vi "FRCts20_Backend_GenerateStats.vi"(8 "error in (no error)":errorcluster, 9 "Key":string, 11 "TeamData":T1) -> (0 "error out":errorcluster)   [LabVIEW 2014, in "FRCts20_Backend_Engine_Deprecated.lvlib"]
uses:
  FRCts20_Backend_Engine_Deprecated.lvlib
  FRCts20_Backend_NumTeams.ctl
  FRCts20_Backend_Controls.lvlib
  FRCts20_Backend_PercTeams.ctl
  FRCts20_Backend_SoftwareUsage.ctl
  FRCts20_Backend_ResPerDayPerQuad.ctl
  FRCts20_Backend_ResDayTotals.ctl
  FRCts20_Backend_ResQuadTotals.ctl
  FRCts20_Backend_Resolved.ctl
  FRCts20_Backend_OpenQuadTotals.ctl
  FRCts20_Backend_Open.ctl
  FRCts20_Backend_Issues.ctl
  FRCts20_Backend_Stats.ctl
  FRCts20_Backend_Engine.lvlib
  FRCts20_Backend_FGVOperation.ctl
  FRCts20_Backend_FGVDatesCommands.ctl
  FRCts20_Backend_IssueDfn.ctl
  FRCts20_Backend_TeamDfn.ctl
  FRCts20_Backend_TeamDataDfn.ctl
  FRCts20_Backend_Team_Info.ctl
  FRCts20_Backend_Note.ctl
  FRCts20_Backend_Note_list.ctl
  FRCts20_Backend_request_info.ctl
  FRCts20_Backend_IssueTeamList.ctl
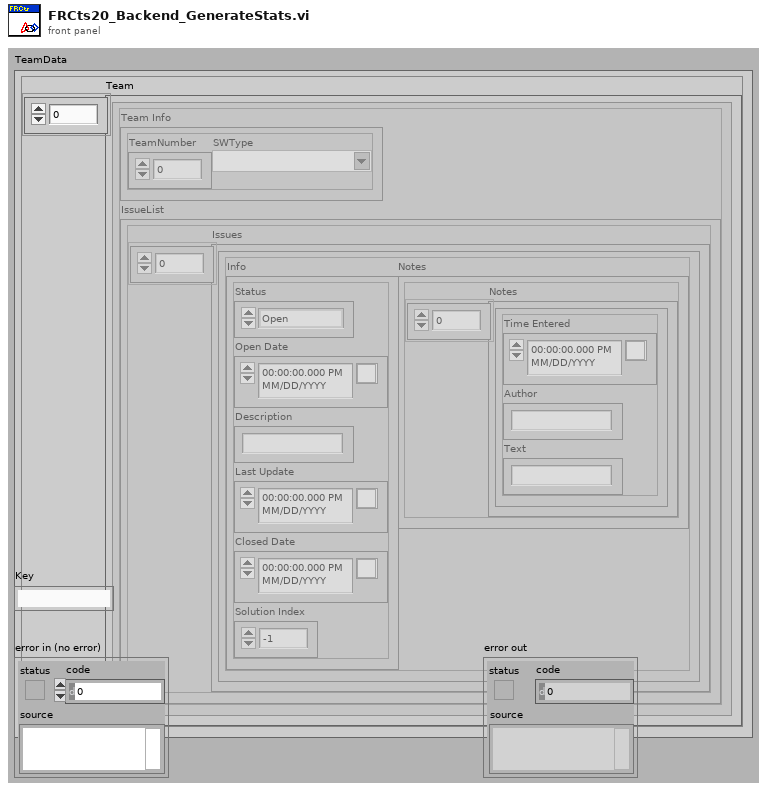
[diagram p1: front panel]
types:
  T1 = typedef "FRCts20_Backend_Controls.lvlib/FRCts20_Backend_TeamDataDfn.ctl" = cluster{"Team":T2[]}
  T2 = typedef "FRCts20_Backend_Controls.lvlib/FRCts20_Backend_TeamDfn.ctl" = cluster{"Team Info":T3, "IssueList":T4}
  T3 = typedef "FRCts20_Backend_Controls.lvlib/FRCts20_Backend_Team_Info.ctl" = cluster{"TeamNumber":u16, "SWType":string}
  T4 = typedef "FRCts20_Backend_Controls.lvlib/FRCts20_Backend_IssueTeamList.ctl" = cluster{"Issues":T5[]}
  T5 = typedef "FRCts20_Backend_Controls.lvlib/FRCts20_Backend_IssueDfn.ctl" = cluster{"Notes":T6, "Info":T8}
  T6 = typedef "FRCts20_Backend_Controls.lvlib/FRCts20_Backend_Note_list.ctl" = cluster{"Notes":T7[]}
  T7 = typedef "FRCts20_Backend_Controls.lvlib/FRCts20_Backend_Note.ctl" = cluster{"Time Entered":timestamp, "Author":string, "Text":string}
  T8 = typedef "FRCts20_Backend_Controls.lvlib/FRCts20_Backend_request_info.ctl" = cluster{"Status":enum16{"Open", "In Work", "Closed"}, "Open Date":timestamp, "Description":string, "Last Update":timestamp, "Closed Date":timestamp, "Solution Index":i32}
  T9 = typedef "FRCts20_Backend_Engine.lvlib/FRCts20_Backend_FGVOperation.ctl" = enum16{"Initialize", "EnqueueMessage", "EnqueueDataReturn", "FlushMessage", "FlushDataReturn"}
  T10 = typedef "FRCts20_Backend_Controls.lvlib/FRCts20_Backend_FGVDatesCommands.ctl" = enum16{"Set Dates", "Get Day", "Get First Day"}
  T11 = typedef "FRCts20_Backend_Controls.lvlib/FRCts20_Backend_Stats.ctl" = cluster{"SoftwareUsage":T12, "Issues":T15}
  T12 = typedef "FRCts20_Backend_Controls.lvlib/FRCts20_Backend_SoftwareUsage.ctl" = cluster{"NumTeams":T13, "PercTeams":T14}
  T13 = typedef "FRCts20_Backend_Controls.lvlib/FRCts20_Backend_NumTeams.ctl" = cluster{"LabVIEW_Num":u16, "C_Cpp_Num":u16, "Java_Num":u16, "Other_Num":u16}
  T14 = typedef "FRCts20_Backend_Controls.lvlib/FRCts20_Backend_PercTeams.ctl" = cluster{"LabVIEW_Perc":dbl, "C_Cpp_Perc":dbl, "Java_Perc":dbl, "Other_Perc":dbl}
  T15 = typedef "FRCts20_Backend_Controls.lvlib/FRCts20_Backend_Issues.ctl" = cluster{"Resolved":T16, "Open":T20}
  T16 = typedef "FRCts20_Backend_Controls.lvlib/FRCts20_Backend_Resolved.ctl" = cluster{"Total":u16, "AvgTimeRes":dbl, "PerDayPerQuad":T17, "DayTotals":T18, "QuadTotals":T19}
  T17 = typedef "FRCts20_Backend_Controls.lvlib/FRCts20_Backend_ResPerDayPerQuad.ctl" = cluster{"Day1Quad1":u16, "Day1Quad2":u16, "Day1Quad3":u16, "Day1Quad4":u16, "Day2Quad1":u16, "Day2Quad2":u16, "Day2Quad3":u16, "Day2Quad4":u16, "Day3Quad1":u16, "Day3Quad2":u16, "Day3Quad3":u16, "Day3Quad4":u16, "Day4Quad1":u16, "Day4Quad2":u16, "Day4Quad3":u16, "Day4Quad4":u16}
  T18 = typedef "FRCts20_Backend_Controls.lvlib/FRCts20_Backend_ResDayTotals.ctl" = cluster{"Day1":u16, "Day2":u16, "Day3":u16, "Day4":u16}
  T19 = typedef "FRCts20_Backend_Controls.lvlib/FRCts20_Backend_ResQuadTotals.ctl" = cluster{"Quad1":u16, "Quad2":u16, "Quad3":u16, "Quad4":u16}
  T20 = typedef "FRCts20_Backend_Controls.lvlib/FRCts20_Backend_Open.ctl" = cluster{"Total":u16, "QuadTotals":T21}
  T21 = typedef "FRCts20_Backend_Controls.lvlib/FRCts20_Backend_OpenQuadTotals.ctl" = cluster{"Quad1":u16, "Quad2":u16, "Quad3":u16, "Quad4":u16}
  T22 = cluster{"LabVIEW_Num":dbl, "C_Cpp_Num":dbl, "Java_Num":dbl, "Other_Num":dbl}
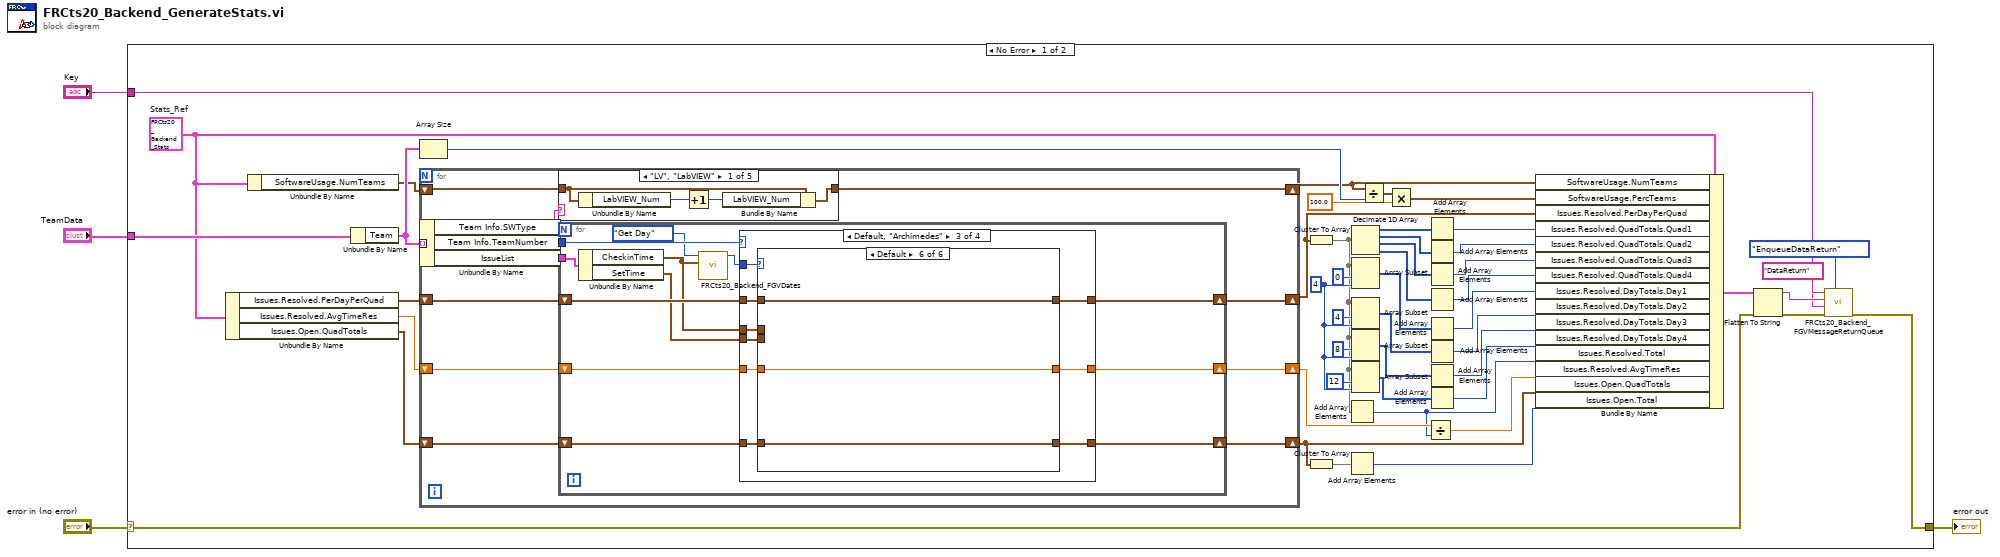
[diagram p0: block diagram]
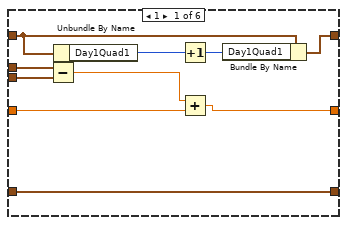
[diagram p3: hidden frame]
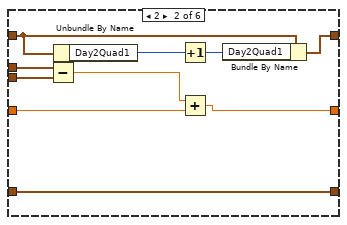
[diagram p4: hidden frame]
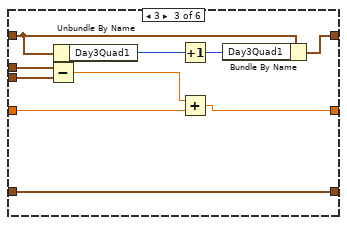
[diagram p5: hidden frame]
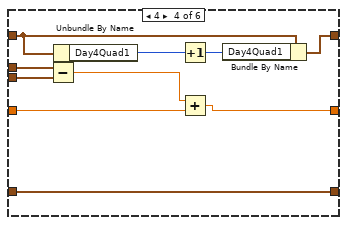
[diagram p6: hidden frame]
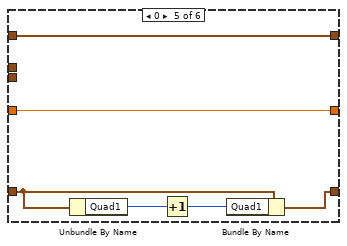
[diagram p7: hidden frame]
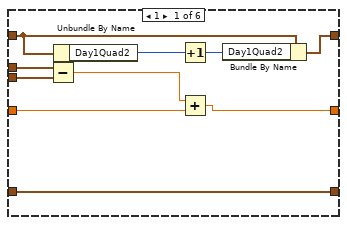
[diagram p9: hidden frame]
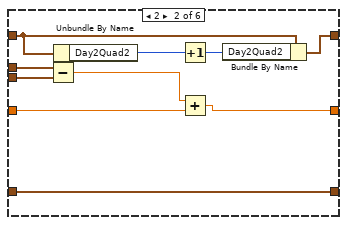
[diagram p10: hidden frame]
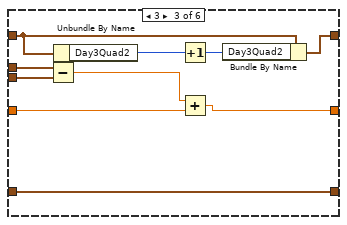
[diagram p11: hidden frame]
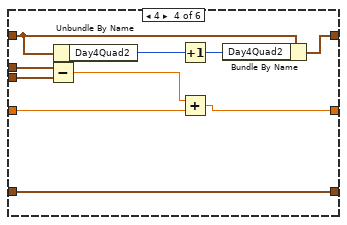
[diagram p12: hidden frame]
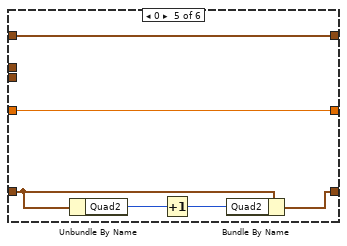
[diagram p13: hidden frame]
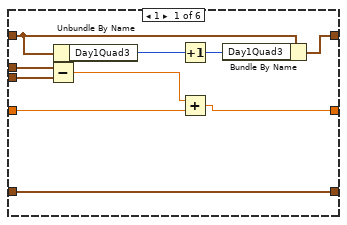
[diagram p14: hidden frame]
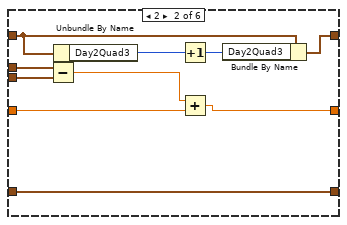
[diagram p15: hidden frame]
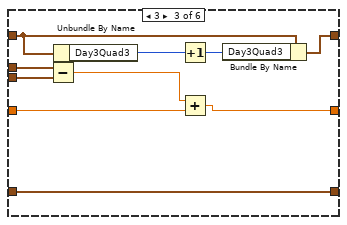
[diagram p16: hidden frame]
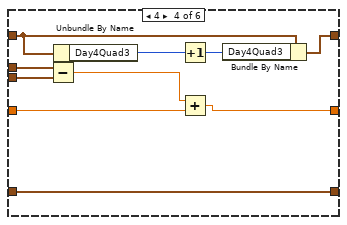
[diagram p17: hidden frame]
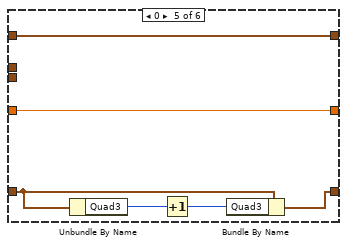
[diagram p18: hidden frame]
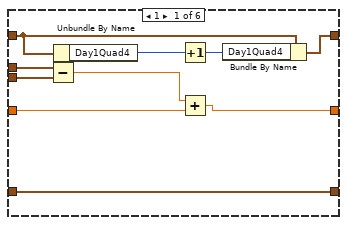
[diagram p20: hidden frame]
diagram:
  n1 = case shown="No Error" "error in (no error)" {
    selector: "error in (no error)" -> [w12 w327]
    tunnel: "TeamData" -> [w53 _]
    tunnel: [w6 w327] -> w2
    tunnel: "Key" -> [w5 _]
    frame No Error {
      w13 = T11 {"SoftwareUsage"={"NumTeams"={"LabVIEW_Num"=0, "C_Cpp_Num"=0, "Java_Num"=0, "Other_Num"=0}, "PercTeams"={"LabVIEW_Perc"=0.0, "C_Cpp_Perc"=0.0, "Java_Perc"=0.0, "Other_Perc"=0.0}}, "Issues"={"Resolved"={"Total"=0, "AvgTimeRes"=0.0, "PerDayPerQuad"={"Day1Quad1"=0, "Day1Quad2"=0, "Day1Quad3"=0, "Day1Quad4"=0, "Day2Quad1"=0, "Day2Quad2"=0, "Day2Quad3"=0, "Day2Quad4"=0, "Day3Quad1"=0, "Day3Quad2"=0, "Day3Quad3"=0, "Day3Quad4"=0, "Day4Quad1"=0, "Day4Quad2"=0, "Day4Quad3"=0, "Day4Quad4"=0}, "DayTotals"={"Day1"=0, "Day2"=0, "Day3"=0, "Day4"=0}, "QuadTotals"={"Quad1"=0, "Quad2"=0, "Quad3"=0, "Quad4"=0}}, "Open"={"Total"=0, "QuadTotals"={"Quad1"=0, "Quad2"=0, "Quad3"=0, "Quad4"=0}}}}  # Stats_Ref
      w35 = 4 ("length")
      n2 = Unbundle By Name(w13) -> ("Issues.Resolved.PerDayPerQuad"=w48:T17, "Issues.Resolved.AvgTimeRes"=w18:dbl, "Issues.Open.QuadTotals"=w19:T21)
      n3 = Unbundle By Name(w13) -> ("SoftwareUsage.NumTeams"=w47:T13)
      n4 = Unbundle By Name(w53) -> ("Team"=w52:T2[])
      n5 = Array Size(array=w52) -> (size(s)=w51:i32)
      n6 = for {
        tunnel: w52 -> [w65] mode=indexing
        shift-right: [w62] -> w46
        shift-left: w47 -> [w63]
        shift-right: [w60] -> w44
        shift-left: w48 -> [w61]
        shift-right: [w54] -> w21
        shift-left: w19 -> [w59]
        shift-right: [w55] -> w16
        shift-left: w18 -> [w56]
        n7 = Unbundle By Name(w65) -> ("Team Info.SWType"=w64:string, "Team Info.TeamNumber"=w57:u16, "IssueList"=w58:T4)
        n8 = case shown="\"LV\", \"LabVIEW\"" w64 {
          tunnel: w63 -> [w313 w314 w318 w322 w326]
          tunnel: [w310 w314 w315 w319 w323] -> w62
          frame "LV", "LabVIEW" {
            n9 = Unbundle By Name(w313) -> ("LabVIEW_Num"=w312:u16)
            n10 = Increment(x=w312) -> (x+1=w311:u16)
            n11 = Bundle By Name(cluster=w313, "LabVIEW_Num"=w311) -> (w310:T13)
          }
          frame Default {
          }
          frame "Other" {
            n12 = Unbundle By Name(w318) -> ("Other_Num"=w317:u16)
            n13 = Increment(x=w317) -> (x+1=w316:u16)
            n14 = Bundle By Name(cluster=w318, "Other_Num"=w316) -> (w315:T13)
          }
          frame "C++", "Windriver, C++" {
            n15 = Unbundle By Name(w322) -> ("C_Cpp_Num"=w321:u16)
            n16 = Increment(x=w321) -> (x+1=w320:u16)
            n17 = Bundle By Name(cluster=w322, "C_Cpp_Num"=w320) -> (w319:T13)
          }
          frame "Java", "JavaBeans" {
            n18 = Unbundle By Name(w326) -> ("Java_Num"=w325:u16)
            n19 = Increment(x=w325) -> (x+1=w324:u16)
            n20 = Bundle By Name(cluster=w326, "Java_Num"=w324) -> (w323:T13)
          }
        }
        n21 = for {
          tunnel: w58 -> [w74]
          shift-right: [w76] -> w60
          shift-left: w61 -> [w77]
          shift-right: [w72] -> w54
          shift-left: w59 -> [w73]
          tunnel: w57 -> [w75]
          shift-right: [w69] -> w55
          shift-left: w56 -> [w70]
          n22 = Unbundle By Name(w74) -> ("CheckinTime"=w67:timestamp, "SetTime"=w71:timestamp)
          n23 = call "FRCts20_Backend_FGVDates.vi"("Date"=w67, "Command"=FRCts20_Backend_FGVDatesCommands."Get Day") -> ("Day"=w68:i32)  [unwired: 7 in, 2 out]
          n24 = case shown="Default, \"Archimedes\"" w75 {
            tunnel: w77 -> [w86 w144 w202 w260]
            tunnel: [w85 w143 w201 w259] -> w76
            tunnel: w73 -> [w84 w142 w200 w258]
            tunnel: [w83 w141 w199 w257] -> w72
            tunnel: w71 -> [w82 w140 w198 w256]
            tunnel: w70 -> [w81 w139 w197 w255]
            tunnel: [w80 w138 w196 w254] -> w69
            tunnel: w67 -> [w79 w137 w195 w253]
            tunnel: w68 -> [w78 w136 w194 w252]
            frame 3 {
              n25 = case shown="Default" w78 {
                tunnel: w86 -> [w96 w106 w116 w126 w132 w135]
                tunnel: [w93 w103 w113 w123 w132 w135] -> w85
                tunnel: w84 -> [w92 w102 w112 w122 w129 w133]
                tunnel: [w92 w102 w112 w122 w128 w133] -> w83
                tunnel: w82 -> [w90 w99 w109 w119 _ _]
                tunnel: w81 -> [w89 w98 w108 w118 w127 w134]
                tunnel: [w87 w97 w107 w117 w127 w134] -> w80
                tunnel: w79 -> [w91 w100 w110 w120 _ _]
                frame 1 {
                  n26 = Subtract(x=w91, y=w90) -> (x-y=w88:dbl)
                  n27 = Unbundle By Name(w96) -> ("Day1Quad1"=w95:u16)
                  n28 = Increment(x=w95) -> (x+1=w94:u16)
                  n29 = Add(x=w88, y=w89) -> (x+y=w87:dbl)
                  n30 = Bundle By Name(cluster=w96, "Day1Quad1"=w94) -> (w93:T17)
                }
                frame 2 {
                  n31 = Subtract(x=w100, y=w99) -> (x-y=w101:dbl)
                  n32 = Unbundle By Name(w106) -> ("Day2Quad1"=w105:u16)
                  n33 = Increment(x=w105) -> (x+1=w104:u16)
                  n34 = Add(x=w101, y=w98) -> (x+y=w97:dbl)
                  n35 = Bundle By Name(cluster=w106, "Day2Quad1"=w104) -> (w103:T17)
                }
                frame 3 {
                  n36 = Subtract(x=w110, y=w109) -> (x-y=w111:dbl)
                  n37 = Unbundle By Name(w116) -> ("Day3Quad1"=w115:u16)
                  n38 = Increment(x=w115) -> (x+1=w114:u16)
                  n39 = Add(x=w111, y=w108) -> (x+y=w107:dbl)
                  n40 = Bundle By Name(cluster=w116, "Day3Quad1"=w114) -> (w113:T17)
                }
                frame 4 {
                  n41 = Subtract(x=w120, y=w119) -> (x-y=w121:dbl)
                  n42 = Unbundle By Name(w126) -> ("Day4Quad1"=w125:u16)
                  n43 = Increment(x=w125) -> (x+1=w124:u16)
                  n44 = Add(x=w121, y=w118) -> (x+y=w117:dbl)
                  n45 = Bundle By Name(cluster=w126, "Day4Quad1"=w124) -> (w123:T17)
                }
                frame 0 {
                  n46 = Unbundle By Name(w129) -> ("Quad1"=w131:u16)
                  n47 = Increment(x=w131) -> (x+1=w130:u16)
                  n48 = Bundle By Name(cluster=w129, "Quad1"=w130) -> (w128:T21)
                }
                frame Default {
                }
              }
            }
            frame 2 {
              n49 = case shown="Default" w136 {
                tunnel: w144 -> [w154 w164 w174 w184 w190 w193]
                tunnel: [w151 w161 w171 w181 w190 w193] -> w143
                tunnel: w142 -> [w150 w160 w170 w180 w187 w191]
                tunnel: [w150 w160 w170 w180 w186 w191] -> w141
                tunnel: w140 -> [w148 w157 w167 w177 _ _]
                tunnel: w139 -> [w147 w156 w166 w176 w185 w192]
                tunnel: [w145 w155 w165 w175 w185 w192] -> w138
                tunnel: w137 -> [w149 w158 w168 w178 _ _]
                frame 1 {
                  n50 = Subtract(x=w149, y=w148) -> (x-y=w146:dbl)
                  n51 = Unbundle By Name(w154) -> ("Day1Quad2"=w153:u16)
                  n52 = Increment(x=w153) -> (x+1=w152:u16)
                  n53 = Add(x=w146, y=w147) -> (x+y=w145:dbl)
                  n54 = Bundle By Name(cluster=w154, "Day1Quad2"=w152) -> (w151:T17)
                }
                frame 2 {
                  n55 = Subtract(x=w158, y=w157) -> (x-y=w159:dbl)
                  n56 = Unbundle By Name(w164) -> ("Day2Quad2"=w163:u16)
                  n57 = Increment(x=w163) -> (x+1=w162:u16)
                  n58 = Add(x=w159, y=w156) -> (x+y=w155:dbl)
                  n59 = Bundle By Name(cluster=w164, "Day2Quad2"=w162) -> (w161:T17)
                }
                frame 3 {
                  n60 = Subtract(x=w168, y=w167) -> (x-y=w169:dbl)
                  n61 = Unbundle By Name(w174) -> ("Day3Quad2"=w173:u16)
                  n62 = Increment(x=w173) -> (x+1=w172:u16)
                  n63 = Add(x=w169, y=w166) -> (x+y=w165:dbl)
                  n64 = Bundle By Name(cluster=w174, "Day3Quad2"=w172) -> (w171:T17)
                }
                frame 4 {
                  n65 = Subtract(x=w178, y=w177) -> (x-y=w179:dbl)
                  n66 = Unbundle By Name(w184) -> ("Day4Quad2"=w183:u16)
                  n67 = Increment(x=w183) -> (x+1=w182:u16)
                  n68 = Add(x=w179, y=w176) -> (x+y=w175:dbl)
                  n69 = Bundle By Name(cluster=w184, "Day4Quad2"=w182) -> (w181:T17)
                }
                frame 0 {
                  n70 = Unbundle By Name(w187) -> ("Quad2"=w189:u16)
                  n71 = Increment(x=w189) -> (x+1=w188:u16)
                  n72 = Bundle By Name(cluster=w187, "Quad2"=w188) -> (w186:T21)
                }
                frame Default {
                }
              }
            }
            frame 0, Default {
              n73 = case shown="Default" w194 {
                tunnel: w202 -> [w212 w222 w232 w242 w248 w251]
                tunnel: [w209 w219 w229 w239 w248 w251] -> w201
                tunnel: w200 -> [w208 w218 w228 w238 w245 w249]
                tunnel: [w208 w218 w228 w238 w244 w249] -> w199
                tunnel: w198 -> [w206 w215 w225 w235 _ _]
                tunnel: w197 -> [w205 w214 w224 w234 w243 w250]
                tunnel: [w203 w213 w223 w233 w243 w250] -> w196
                tunnel: w195 -> [w207 w216 w226 w236 _ _]
                frame 1 {
                  n74 = Subtract(x=w207, y=w206) -> (x-y=w204:dbl)
                  n75 = Unbundle By Name(w212) -> ("Day1Quad3"=w211:u16)
                  n76 = Increment(x=w211) -> (x+1=w210:u16)
                  n77 = Add(x=w204, y=w205) -> (x+y=w203:dbl)
                  n78 = Bundle By Name(cluster=w212, "Day1Quad3"=w210) -> (w209:T17)
                }
                frame 2 {
                  n79 = Subtract(x=w216, y=w215) -> (x-y=w217:dbl)
                  n80 = Unbundle By Name(w222) -> ("Day2Quad3"=w221:u16)
                  n81 = Increment(x=w221) -> (x+1=w220:u16)
                  n82 = Add(x=w217, y=w214) -> (x+y=w213:dbl)
                  n83 = Bundle By Name(cluster=w222, "Day2Quad3"=w220) -> (w219:T17)
                }
                frame 3 {
                  n84 = Subtract(x=w226, y=w225) -> (x-y=w227:dbl)
                  n85 = Unbundle By Name(w232) -> ("Day3Quad3"=w231:u16)
                  n86 = Increment(x=w231) -> (x+1=w230:u16)
                  n87 = Add(x=w227, y=w224) -> (x+y=w223:dbl)
                  n88 = Bundle By Name(cluster=w232, "Day3Quad3"=w230) -> (w229:T17)
                }
                frame 4 {
                  n89 = Subtract(x=w236, y=w235) -> (x-y=w237:dbl)
                  n90 = Unbundle By Name(w242) -> ("Day4Quad3"=w241:u16)
                  n91 = Increment(x=w241) -> (x+1=w240:u16)
                  n92 = Add(x=w237, y=w234) -> (x+y=w233:dbl)
                  n93 = Bundle By Name(cluster=w242, "Day4Quad3"=w240) -> (w239:T17)
                }
                frame 0 {
                  n94 = Unbundle By Name(w245) -> ("Quad3"=w247:u16)
                  n95 = Increment(x=w247) -> (x+1=w246:u16)
                  n96 = Bundle By Name(cluster=w245, "Quad3"=w246) -> (w244:T21)
                }
                frame Default {
                }
              }
            }
            frame 1 {
              n97 = case shown="Default" w252 {
                tunnel: w260 -> [w270 w280 w290 w300 w306 w309]
                tunnel: [w267 w277 w287 w297 w306 w309] -> w259
                tunnel: w258 -> [w266 w276 w286 w296 w303 w307]
                tunnel: [w266 w276 w286 w296 w302 w307] -> w257
                tunnel: w256 -> [w264 w273 w283 w293 _ _]
                tunnel: w255 -> [w263 w272 w282 w292 w301 w308]
                tunnel: [w261 w271 w281 w291 w301 w308] -> w254
                tunnel: w253 -> [w265 w274 w284 w294 _ _]
                frame 1 {
                  n98 = Subtract(x=w265, y=w264) -> (x-y=w262:dbl)
                  n99 = Unbundle By Name(w270) -> ("Day1Quad4"=w269:u16)
                  n100 = Increment(x=w269) -> (x+1=w268:u16)
                  n101 = Add(x=w262, y=w263) -> (x+y=w261:dbl)
                  n102 = Bundle By Name(cluster=w270, "Day1Quad4"=w268) -> (w267:T17)
                }
                frame 2 {
                  n103 = Subtract(x=w274, y=w273) -> (x-y=w275:dbl)
                  n104 = Unbundle By Name(w280) -> ("Day2Quad4"=w279:u16)
                  n105 = Increment(x=w279) -> (x+1=w278:u16)
                  n106 = Add(x=w275, y=w272) -> (x+y=w271:dbl)
                  n107 = Bundle By Name(cluster=w280, "Day2Quad4"=w278) -> (w277:T17)
                }
                frame 3 {
                  n108 = Subtract(x=w284, y=w283) -> (x-y=w285:dbl)
                  n109 = Unbundle By Name(w290) -> ("Day3Quad4"=w289:u16)
                  n110 = Increment(x=w289) -> (x+1=w288:u16)
                  n111 = Add(x=w285, y=w282) -> (x+y=w281:dbl)
                  n112 = Bundle By Name(cluster=w290, "Day3Quad4"=w288) -> (w287:T17)
                }
                frame 4 {
                  n113 = Subtract(x=w294, y=w293) -> (x-y=w295:dbl)
                  n114 = Unbundle By Name(w300) -> ("Day4Quad4"=w299:u16)
                  n115 = Increment(x=w299) -> (x+1=w298:u16)
                  n116 = Add(x=w295, y=w292) -> (x+y=w291:dbl)
                  n117 = Bundle By Name(cluster=w300, "Day4Quad4"=w298) -> (w297:T17)
                }
                frame 0 {
                  n118 = Unbundle By Name(w303) -> ("Quad4"=w305:u16)
                  n119 = Increment(x=w305) -> (x+1=w304:u16)
                  n120 = Bundle By Name(cluster=w303, "Quad4"=w304) -> (w302:T21)
                }
                frame Default {
                }
              }
            }
          }
        }
      }
      n121 = Cluster To Array(cluster=w44) -> (array=w17:u16[])
      n122 = Cluster To Array(cluster=w21) -> (array=w22:u16[])
      n123 = Add Array Elements(numeric array=w17) -> (sum=w15:u16)
      n124 = Add Array Elements(numeric array=w22) -> (sum=w20:u16)
      n125 = Decimate 1D Array(w17) -> (w43:u16[], w42:u16[], w41:u16[], w40:u16[])
      n126 = Array Subset(array=w17, index=0, length=w35) -> (w30:u16[])
      n127 = Array Subset(array=w17, index=4, length=w35) -> (w29:u16[])
      n128 = Array Subset(array=w17, index=8, length=w35) -> (w28:u16[])
      n129 = Array Subset(array=w17, index=12, length=w35) -> (w27:u16[])
      n130 = Divide(x=w46, y=w51) -> (x/y=w49:T22)
      n131 = Multiply(x=w49, y=100.0) -> (x*y=w45:T22)
      n132 = Divide(x=w16, y=w15) -> (x/y=w14:dbl)
      n133 = Add Array Elements(numeric array=w43) -> (sum=w39:u16)
      n134 = Add Array Elements(numeric array=w42) -> (sum=w38:u16)
      n135 = Add Array Elements(numeric array=w41) -> (sum=w37:u16)
      n136 = Add Array Elements(numeric array=w40) -> (sum=w36:u16)
      n137 = Add Array Elements(numeric array=w30) -> (sum=w26:u16)
      n138 = Add Array Elements(numeric array=w29) -> (sum=w23:u16)
      n139 = Add Array Elements(numeric array=w28) -> (sum=w24:u16)
      n140 = Add Array Elements(numeric array=w27) -> (sum=w25:u16)
      n141 = Bundle By Name(cluster=w13, "SoftwareUsage.NumTeams"=w46, "SoftwareUsage.PercTeams"=w45, "Issues.Resolved.PerDayPerQuad"=w44, "Issues.Resolved.QuadTotals.Quad1"=w39, "Issues.Resolved.QuadTotals.Quad2"=w38, "Issues.Resolved.QuadTotals.Quad3"=w37, "Issues.Resolved.QuadTotals.Quad4"=w36, "Issues.Resolved.DayTotals.Day1"=w26, "Issues.Resolved.DayTotals.Day2"=w23, "Issues.Resolved.DayTotals.Day3"=w24, "Issues.Resolved.DayTotals.Day4"=w25, "Issues.Resolved.Total"=w15, "Issues.Resolved.AvgTimeRes"=w14, "Issues.Open.QuadTotals"=w21, "Issues.Open.Total"=w20) -> (w11:T11)
      n142 = Flatten To String(anything=w11, error in (no error)=w12) -> (data string=w9:string, error out=w7:errorcluster)  [unwired: 2 in, 1 out]
      n143 = call "FRCts20_Backend_FGVMessageReturnQueue.vi"("Operation"=FRCts20_Backend_FGVOperation."EnqueueDataReturn", "error in (no error)"=w7, "Key"=w5, "Message Value"=w9, "Message Name"="DataReturn") -> ("error out"=w6:errorcluster)  [unwired: 3 in, 1 out]
    }
    frame Error {
    }
  }
  "error out" <- w2
